vi "onTestExecution.vi"(7 "Name":string, 8 "error in (no error)":errorcluster, 11 "Test Runner.Project in":refnum<class "Test Runner.Project.lvclass">) -> (0 "error out":errorcluster, 3 "Test Runner.Project out":refnum<class "Test Runner.Project.lvclass">)   [LabVIEW 2013, in "Caraya.lvlib" / "Test Runner.Project.lvclass"]
uses:
  Test Runner.Project.lvclass
  Test Runner/Test Runner.lvclass
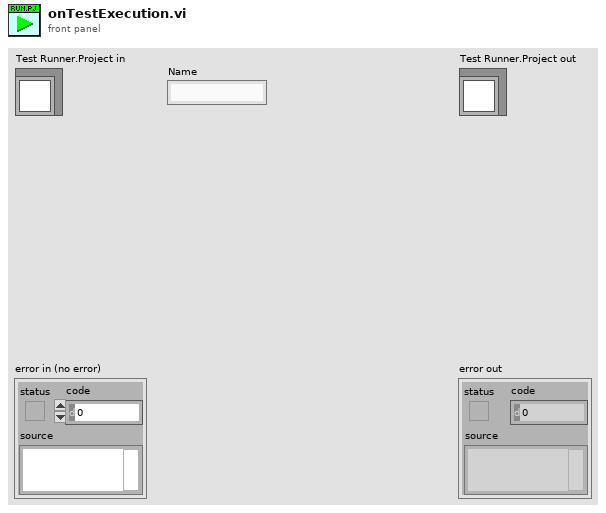
[diagram p1: front panel]
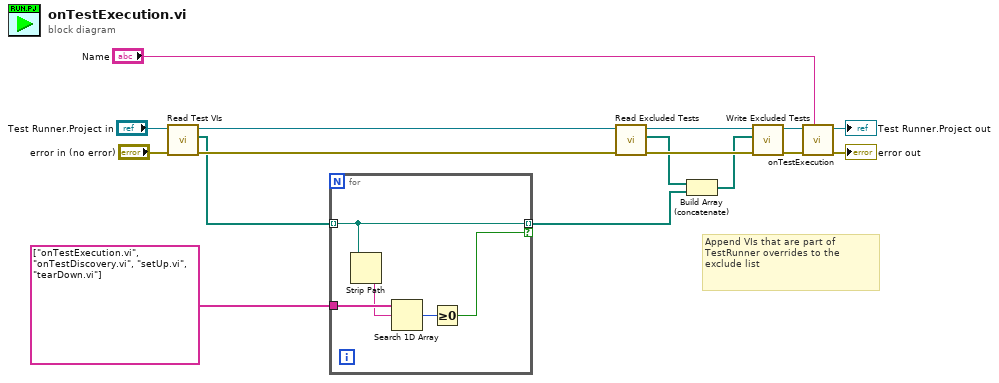
[diagram p0: block diagram]
diagram:
  # "Append VIs that are part of TestRunner overrides to the exclude list"
  n1 = call "Read Test VIs.vi"("error in (no error)"="error in (no error)", "Test Runner in"="Test Runner.Project in") -> ("error out"=w6:errorcluster, "Test VIs"=w3:path[], "Test Runner out"=w8:refnum<class "Test Runner.Project.lvclass">)  [unwired: 7 in]
  n2 = for {
    tunnel: w3 -> [w21] mode=indexing
    tunnel: [w21] -> w2 mode=indexing if=w17
    tunnel: string[] ["onTestExecution.vi", "onTestDiscovery.vi", "setUp.vi", "tearDown.vi"] -> [w20]
    n3 = Strip Path(path=w21) -> (name=w19:string)  [unwired: 1 out]
    n4 = Search 1D Array(1D array=w20, element=w19) -> (index of element=w18:i32)  [unwired: 1 in]
    n5 = Greater Or Equal To 0?(x=w18) -> (x >= 0?=w17:bool)
  }
  n6 = call "Read Excluded Tests.vi"("error in (no error)"=w6, "Test Runner in"=w8) -> ("error out"=w13:errorcluster, "Excluded Tests"=w5:path[], "Test Runner out"=w11:refnum<class "Test Runner.Project.lvclass">)  [unwired: 7 in]
  n7 = Build Array (concatenate)(w5, w2) -> (w4:path[])
  n8 = call "Write Excluded Tests.vi"("error in (no error)"=w13, "Excluded Tests"=w4, "Test Runner in"=w11) -> ("error out"=w12:errorcluster, "Test Runner out"=w10:refnum<class "Test Runner.Project.lvclass">)  [unwired: 7 in]
  n9 = call-parent "onTestExecution.vi"("Name"="Name", "error in (no error)"=w12, "Test Runner in"=w10) -> ("error out"=→"error out":errorcluster, "Test Runner out"=→"Test Runner.Project out":refnum<class "Test Runner.Project.lvclass">)  [unwired: 7 in]
